vi "Coil Get Mapping.vi"(8 "error in (no error)":errorcluster, 11 "Item Ref in":T1 format="%.0x") -> (0 "error out":errorcluster, 2 "Mapping":T2 {"VS Reference" format="%.0x"}, 3 "Item Ref out":T1 format="%.0x")   [LabVIEW 2015]
uses:
  Shared/Controls/Data Model/DataType.ctl
  Shared/Modbus Master Shared.lvlib
  Shared/Controls/Data Model/Mapping.ctl
  <vilib>/NI Veristand/Custom Device API/Custom Device Item Ref.ctl
  <vilib>/NI VeriStand/Custom Device API/Custom Device API.lvlib
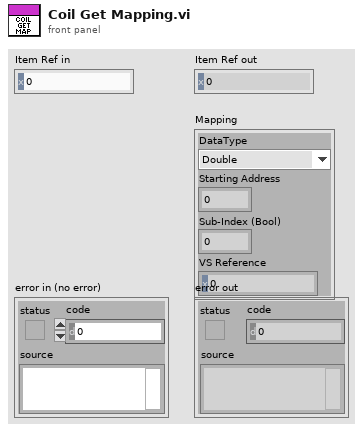
[diagram p1: front panel]
types:
  T1 = typedef "Custom Device API.lvlib/Custom Device Item Ref.ctl" = u64
  T2 = typedef "Modbus Master Shared.lvlib/Mapping.ctl" = cluster{"DataType":T3, "Starting Address":u16, "Sub-Index (Bool)":u16, "VS Reference":T1}
  T3 = typedef "Modbus Master Shared.lvlib/DataType.ctl" = enum16{"Double", "Single", "I64", "I32", "I16", "I8", "U64", "U32", "U16", "U8", "Boolean"}
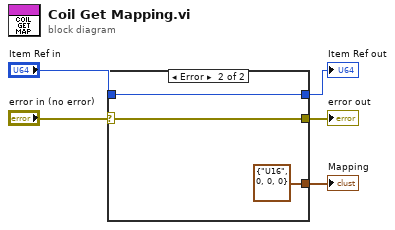
[diagram p0: block diagram]
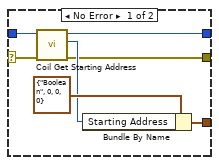
[diagram p2: hidden frame]
diagram:
  n1 = case shown="Error" "error in (no error)" {
    selector: "error in (no error)" -> [w8 w14]
    tunnel: "Item Ref in" -> [w10 w15]
    tunnel: [w9 T2 {"DataType"=enum."U16", "Starting Address"=0, "Sub-Index (Bool)"=0, "VS Reference"=0} ("Mapping")] -> w4
    tunnel: [w7 w14] -> w2
    tunnel: [w6 w15] -> w1
    frame No Error {
      n2 = call "Coil Get Starting Address.vi"("error in (no error)"=w8, "Item Ref in"=w10) -> ("error out"=w7:errorcluster, "Starting Address"=w11:u16, "Item Ref out"=w6:T1)  [unwired: 7 in]
      n3 = Bundle By Name(cluster=T2 {"DataType"=enum."Boolean", "Starting Address"=0, "Sub-Index (Bool)"=0, "VS Reference"=0} ("Mapping"), "Starting Address"=w11) -> (w9:T2)
    }
    frame Error {
    }
  }
  "Mapping" <- w4
  "error out" <- w2
  "Item Ref out" <- w1
